vi "new copy speed test.vi"() -> ()   [LabVIEW 2020, in "Data.PG.lvclass"]
uses:
  Data.PG.lvclass
panel:
  in  "path okay for temporary file":path=path "C:/Users/Phil/Desktop"
  in  "password":string="711elvis"
  in  "username":string="phil"
  in  "table":string="twenty_doubes"
  in  "Path to data csv":path=path "C:/Users/Phil/Desktop/jack/data_speed_test.csv"
  out "Time (ms)":u32
  # "Just put any old path down that labview can write a temporary file to"
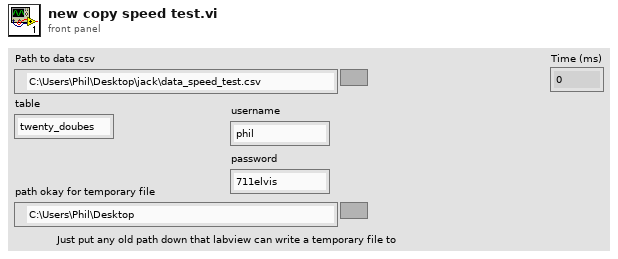
[diagram p1: front panel]
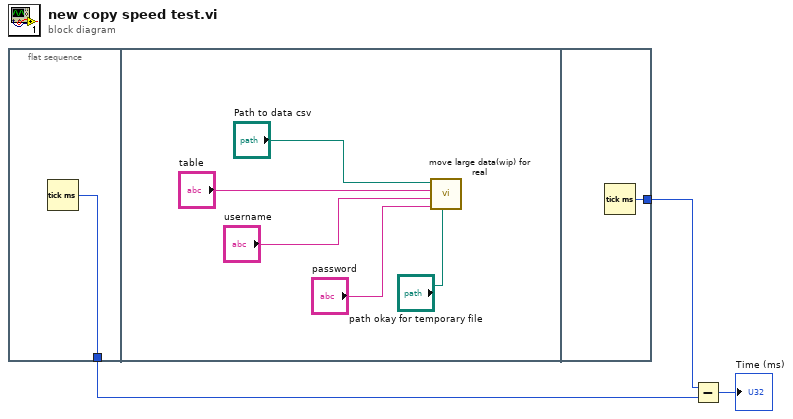
[diagram p0: block diagram]
diagram:
  n1 = flat-sequence {
    tunnel: [w4] -> w2
    tunnel: [w10] -> w3
    frame #0 {
      n2 = Tick Count (ms)() -> (millisecond timer value=w4:u32)
    }
    frame #1 {
      n3 = call "move large data(wip) for real.vi"(6:"path okay for temporary file", 8:"password", 9:"username", 10:"table", 11:"Path to data csv") -> ()  [unwired: 7 in]
    }
    frame #2 {
      n4 = Tick Count (ms)() -> (millisecond timer value=w10:u32)
    }
  }
  n5 = Subtract(x=w3, y=w2) -> (x-y=→"Time (ms)":u32)
